vi "SendMessage.vi"(5 "atributes":variant, 6 "timeout in ms (-1)":i32=-1, 7 "urgent? (F)":bool, 8 "error in":errorcluster, 9 "data":variant, 10 "name":string, 11 "message ref in":refnum<class "CLM_LocalMessage_UserEvent.lvclass">) -> (0 "error out":errorcluster, 3 "message ref out":refnum<class "CLM_LocalMessage_UserEvent.lvclass">, 4 "timed out?":bool)   [LabVIEW 2013, in "CLM_LocalMessage_UserEvent.lvclass"]
uses:
  CLM_LocalMessage_UserEvent.lvclass
  CLM_LocalMessage_UserEvent.lvclass/CLM_LocalMessage_UserEvent.ctl
  LocalMessage/BundleMessageCluster.vi
  SendUserEventMessage_Cluster.vi
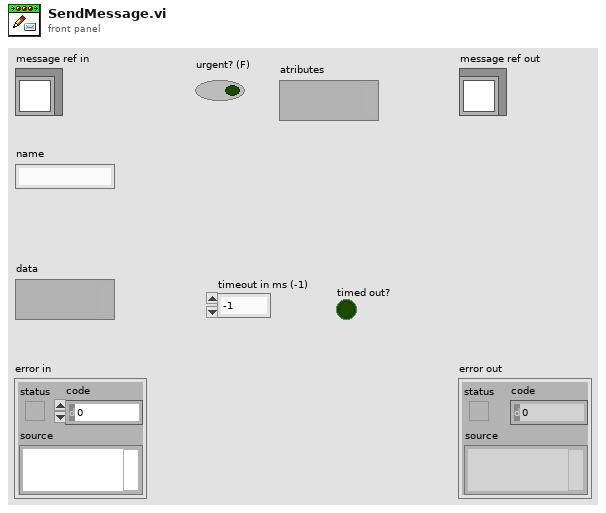
[diagram p1: front panel]
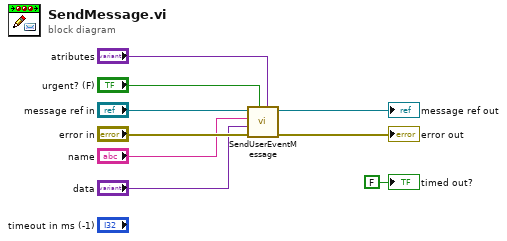
[diagram p0: block diagram]
diagram:
  n1 = call "SendUserEventMessage.vi"("atributes"="atributes", "urgent? (F)"="urgent? (F)", "error in"="error in", "data"="data", "name"="name", "message ref in"="message ref in") -> ("error out"=→"error out":errorcluster, "message ref out"=→"message ref out":refnum<class "CLM_LocalMessage_UserEvent.lvclass">)  [unwired: 4 in]
  "timed out?" <- FALSE ("timed out?")
